vi "Check Error Warnings.vi"(8 "error in (no error)":errorcluster, 11 "Errors to Change to Warning":i32[](array[numeric])=[0, 0, 0, 0]) -> (0 "error out":errorcluster, 3 "Warnings out":bool[](array[boolean]))   [LabVIEW 2018]
doc: "Checks the input error for warning codes and removes the error if found."
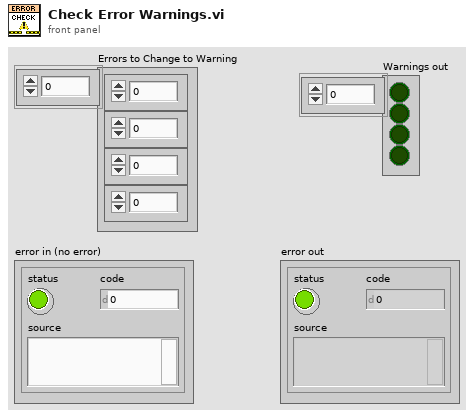
[diagram p1: front panel]
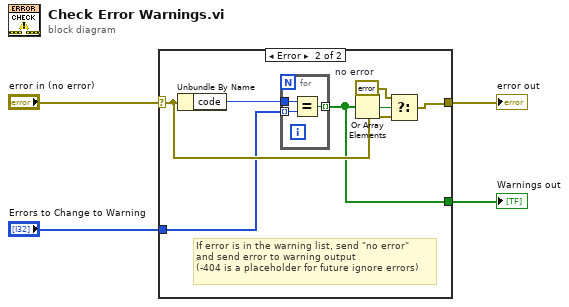
[diagram p0: block diagram]
diagram:
  n1 = case shown="Error" "error in (no error)" {
    selector: "error in (no error)" -> [w5 w9]
    tunnel: [w5 w11] -> w2
    tunnel: [_ w7] -> w3
    tunnel: "Errors to Change to Warning" -> [_ w6]
    frame No Error {
    }
    frame Error {
      w12 = errorcluster {"status"=FALSE, "code"=0, "source"=""}  # no error
      # "If error is in the warning list, send \"no error\"\nand send error to warning output\n(-404 is a placeholder for future ignore errors)"
      n2 = Unbundle By Name(w9) -> ("code"=w8:i32)
      n3 = for {
        tunnel: w6 -> [w14] mode=indexing
        tunnel: w8 -> [w15]
        tunnel: [w13] -> w7 mode=indexing
        n4 = Equal?(x=w15, y=w14) -> (x = y?=w13:bool)
      }
      n5 = Or Array Elements(Boolean array=w7) -> (logical OR=w10:bool)
      n6 = Select(t=w12, s=w10, f=w9) -> (s? t:f=w11:errorcluster)
    }
  }
  "Warnings out" <- w3
  "error out" <- w2
